vi "E7_28_check.vi"(0 "DriverConnect in":T1={"InterfaceType"=enum."VISA", "OpenedSession"="", "InterfaceSettings"={"Interface"=enum."RS232", "EOS 4 read"=enum."LF (\\n)", "EOS 4 write"=enum."LF (\\n)", "TMO, ms"=10000, "Sett"=variant(cluster{"Baud Rate":u32, "Data Bits":u16, "Parity":u16, "Stop Bits":u16, "Flow Control":u16, "Eho":bool} {"Baud Rate"=75, "Data Bits"=0, "Parity"=0, "Stop Bits"=0, "Flow Control"=0, "Eho"=FALSE})}}, 1 "String in":T8, 2 "command string in":T8, 3 "command HEX in":T7, 11 "error in":T9, 13 "Driver Name":T6, 14 "Error Code":T7) -> (4 "DriverConnect out":T1={"InterfaceType"=enum."VISA", "OpenedSession"="", "InterfaceSettings"={"Interface"=enum."RS232", "EOS 4 read"=enum."LF (\\n)", "EOS 4 write"=enum."LF (\\n)", "TMO, ms"=10000, "Sett"=variant(cluster{"Baud Rate":u32, "Data Bits":u16, "Parity":u16, "Stop Bits":u16, "Flow Control":u16, "Eho":bool} {"Baud Rate"=75, "Data Bits"=0, "Parity"=0, "Stop Bits"=0, "Flow Control"=0, "Eho"=FALSE})}}, 15 "error out":T9)   [LabVIEW 2018]
uses:
  MOKO_LabViewLibrary/MokoLowLevel/MokoLowLovelControl/MLLC_Error.ctl
  MOKO_LabViewLibrary/MokoLowLevel/MokoLowLovelControl/MLLC_Command.ctl
  MOKO_LabViewLibrary/MokoLowLevel/MokoLowLovelControl/MLLC_ErrorCode.ctl
  MOKO_LabViewLibrary/MokoLowLevel/MokoLowLovelControl/MLLC_DriverName.ctl
  MOKO_LabViewLibrary/MokoLowLevel/MokoLowLovelControl/MLLC_ConnectCluster.ctl
  MOKO_LabViewLibrary/MokoLowLevel/MokoLowLovelControl/MLLC_InterfaceType.ctl
  MOKO_LabViewLibrary/MokoLowLevel/MokoLowLovelControl/MLLC_OpenedSession.ctl
  MOKO_LabViewLibrary/MokoLowLevel/MokoLowLovelControl/MLLC_InterfaceSettings.ctl
  MOKO_LabViewLibrary/MokoLowLevel/MokoLowLovelControl/MLLC_InterfaceKind.ctl
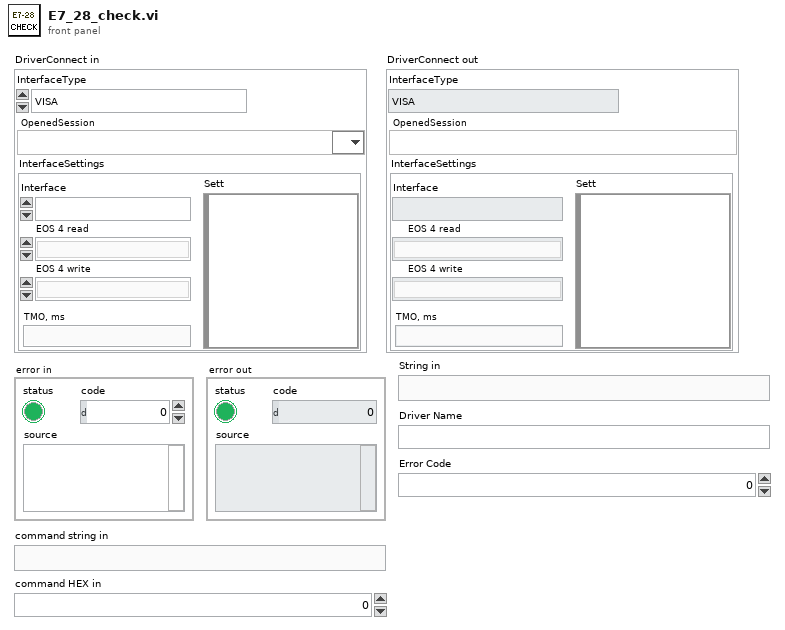
[diagram p1: front panel]
types:
  T1 = typedef "MLLC_ConnectCluster.ctl" = cluster{"InterfaceType":T2, "OpenedSession":T3, "InterfaceSettings":T4}
  T2 = typedef "MLLC_InterfaceType.ctl" = enum16{"VISA", "Prologix USB-GPIB"}
  T3 = typedef "MLLC_OpenedSession.ctl" = refnum<visa-resource-name>
  T4 = typedef "MLLC_InterfaceSettings.ctl" = cluster{"Interface":T5, "EOS 4 read":enum16{"Default (=EOS 4 write)", "CR (\\r)", "LF (\\n)", "None"}, "EOS 4 write":enum16{"CR+LF (\\r\\n)", "CR (\\r)", "LF (\\n)", "None"}, "TMO, ms":i32, "Sett":variant}
  T5 = typedef "MLLC_InterfaceKind.ctl" = enum16{"RS232", "GPIB", "USB", "Ethernet", "another"}
  T6 = typedef "MLLC_DriverName.ctl" = string
  T7 = typedef "MLLC_ErrorCode.ctl" = u32
  T8 = typedef "MLLC_Command.ctl" = string
  T9 = typedef "MLLC_Error.ctl" = errorcluster
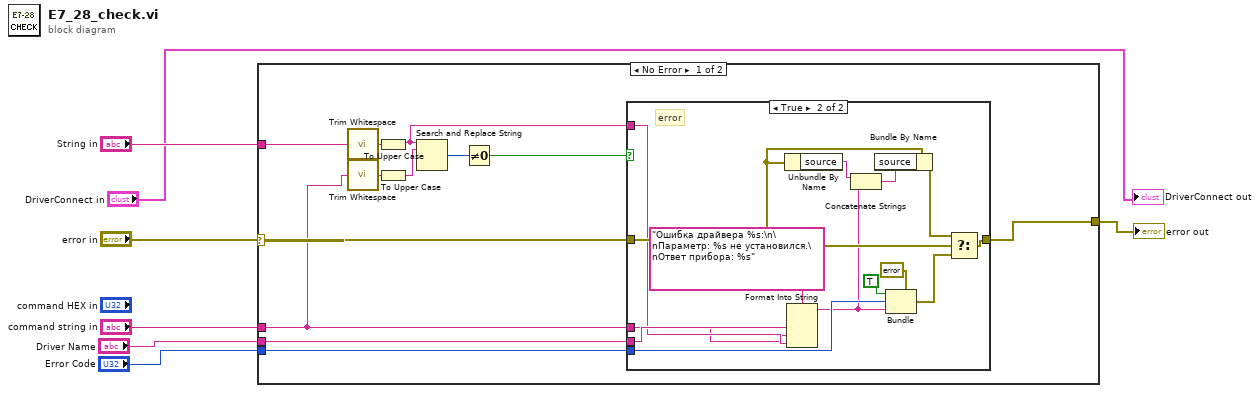
[diagram p0: block diagram]
diagram:
  n1 = case shown="No Error" "error in" {
    selector: "error in" -> [w16 w35]
    tunnel: [w12 w35] -> w7
    tunnel: "String in" -> [w10 _]
    tunnel: "command string in" -> [w11 _]
    tunnel: "Error Code" -> [w14 _]
    tunnel: "Driver Name" -> [w13 _]
    frame No Error {
      n2 = call <vilib>:"Trim Whitespace.vi"("string"=w10) -> ("trimmed string"=w19:string)  [unwired: 1 in]
      n3 = call <vilib>:"Trim Whitespace.vi"("string"=w11) -> ("trimmed string"=w18:string)  [unwired: 1 in]
      n4 = To Upper Case(1:w19) -> (0:w15:string)
      n5 = To Upper Case(1:w18) -> (0:w17:string)
      n6 = Search and Replace String(input string=w15, search string=w17) -> (number of replacements=w9:i32)  [unwired: 6 in, 3 out]
      n7 = Not Equal To 0?(x=w9) -> (x != 0?=w8:bool)
      n8 = case shown="True" w8 {
        tunnel: [w20 w24] -> w12
        tunnel: w16 -> [w20 w30]
        tunnel: w15 -> [_ w22]
        tunnel: w14 -> [_ w31]
        tunnel: w11 -> [_ w21]
        tunnel: w13 -> [_ w23]
        frame False {
          # "no error"
        }
        frame True {
          # "error"
          n9 = Unbundle By Name(w30) -> ("source"=w29:string)
          n10 = Format Into String(format string="Ошибка драйвера %s:\n\nПараметр: %s не установился.\nОтвет прибора: %s", w23, w21, w22) -> (resulting string=w27:string)  [unwired: 2 in, 1 out]
          n11 = Concatenate Strings(w29, w27) -> (w28:string)
          n12 = Bundle By Name(cluster=w30, "source"=w28) -> (w26:errorcluster)
          n13 = Bundle(cluster=errorcluster {"status"=FALSE, "code"=0, "source"=""} ("error out"), "status"=TRUE ("Status"), "code"=w31, "source"=w27) -> (w25:errorcluster)
          n14 = Select(t=w26, s=w30, f=w25) -> (s? t:f=w24:errorcluster)
        }
      }
    }
    frame Error {
    }
  }
  "error out" <- w7
  "DriverConnect out" <- "DriverConnect in"
